vi "Pcre2GetMatchOffsetsFromMatchResult8.vi"(8 "error in":errorcluster, 10 "MatchResult":i32=-1, 11 "pMatchData":u64 format="%.0x") -> (0 "error out":errorcluster, 1 "OffsetsPastMatch":i32[](array[numeric]), 2 "MatchOffsets":i32[](array[numeric]), 3 "pMatchData":u64 format="%.0x")   [LabVIEW 2021, in "libpcre2-8.lvlib"]
uses:
  libpcre2-8.lvlib
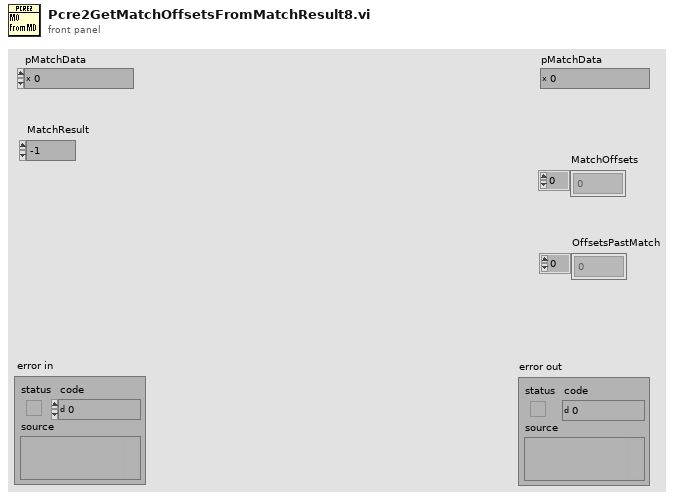
[diagram p1: front panel]
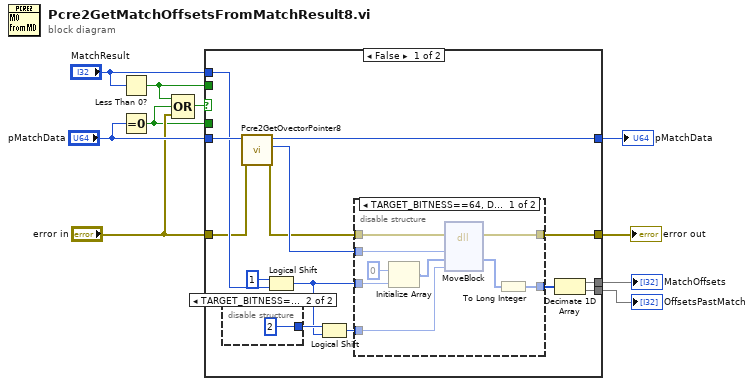
[diagram p0: block diagram]
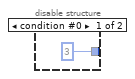
[diagram p2: hidden frame]
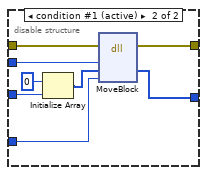
[diagram p3: hidden frame]
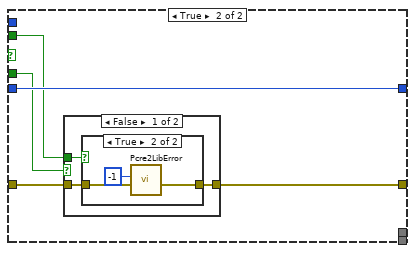
[diagram p4: hidden frame]
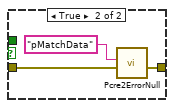
[diagram p6: hidden frame]
diagram:
  n1 = Less Than 0?(x="MatchResult") -> (x < 0?=w2:bool)
  n2 = Equal To 0?(x="pMatchData") -> (x = 0?=w1:bool)
  n3 = Compound Arithmetic op=OR(w2, w1, "error in") -> (w5:bool)
  n4 = case shown="False" w5 {
    tunnel: "error in" -> [w12 w45]
    tunnel: [w24 w47] -> w10
    tunnel: "pMatchData" -> [w20 w48]
    tunnel: [w13 w48] -> w9
    tunnel: [w22 _] -> w7
    tunnel: [w21 _] -> w6
    tunnel: "MatchResult" -> [w18 _]
    tunnel: w2 -> [_ w44]
    tunnel: w1 -> [_ w46]
    frame False {
      n5 = disable-structure shown="TARGET_BITNESS==32" {
        disable-tunnel: [i16 3 ("y") i16 2 ("y")] -> w15
        frame condition #0 {
        }
        frame condition #1 (active) {
        }
      }
      n6 = call "Pcre2GetOvectorPointer8.vi"("error in"=w12, "pMatchData"=w20) -> ("error out"=w11:errorcluster, "pOvector"=w19:u64, "pMatchData"=w13:u64)  [unwired: 7 in]
      n7 = Logical Shift(y=i16 1, x=w18) -> (x << y=w14:i32)
      n8 = Logical Shift(y=w15, x=w14) -> (x << y=w16:i32)
      n9 = disable-structure shown="TARGET_BITNESS==64, Default" {
        disable-tunnel: w19 -> [w35 w43]
        disable-tunnel: [w34 w42] -> w24
        disable-tunnel: w11 -> [w33 w41]
        disable-tunnel: w16 -> [w31 w39]
        disable-tunnel: w14 -> [w30 w38]
        disable-tunnel: [w27 w36] -> w23
        frame condition #0 {
          n10 = Initialize Array(i64 0 ("element"), w30) -> (w29:i64[])
          n11 = dll-call lib="LabVIEW" fn="MoveBlock"(error in=w33, "pointerSrc"=w35, "pointerDest"=w29, "size"=w31) -> (error out=w34:errorcluster, "pointerDest"=w28:i64[])  [unwired: 5 in, 1 out]
          n12 = To Long Integer(number=w28) -> (32bit integer=w27:i32[])
        }
        frame condition #1 (active) {
          n13 = Initialize Array(0 ("element"), w38) -> (w37:i32[])
          n14 = dll-call lib="LabVIEW" fn="MoveBlock"(error in=w41, "pointerSrc"=w43, "pointerDest"=w37, "size"=w39) -> (error out=w42:errorcluster, "pointerDest"=w36:i32[])  [unwired: 5 in, 1 out]
        }
      }
      n15 = Decimate 1D Array(w23) -> (w22:i32[], w21:i32[])
    }
    frame True {
      n16 = case shown="False" w46 {
        tunnel: w45 -> [w50 w57]
        tunnel: [w49 w56] -> w47
        tunnel: w44 -> [w51 _]
        frame False {
          n17 = case shown="True" w51 {
            tunnel: w50 -> [w52 w55]
            tunnel: [w52 w54] -> w49
            frame False {
            }
            frame True {
              n18 = call "Pcre2LibError.vi"("error in"=w55, "ErrorCode"=-1) -> ("error out"=w54:errorcluster)  [unwired: 9 in]
            }
          }
        }
        frame True {
          n19 = call "Pcre2ErrorNull.vi"("error in"=w57, "What"="pMatchData") -> ("error out"=w56:errorcluster)  [unwired: 9 in]
        }
      }
    }
  }
  "pMatchData" <- w9
  "error out" <- w10
  "MatchOffsets" <- w7
  "OffsetsPastMatch" <- w6
